vi "dfd_FXP Direct FIR with IS.vi"(6 "state in":i64[](array[numeric]), 7 "FXPOPs":T5[](array[typedef]) {"source" items=["Coef a/k"=0, "Coef b/v"=7, "Input"=1, "Output"=2, "Multiplicand"=3, "Product"=4, "Sum"=5, "Delay"=6, "Gain"=8]}, 8 "filtering statistics in":T4(array[cluster]) {"statistics information"."min value" format="%.2f"; "statistics information"."max value" format="%.2f"; "Quantizer Source" items=["Coefficients a/k"=0, "Coefficients b/v"=7, "Input"=1, "Output"=2, "Multiplicand"=3, "Product"=4, "Sum"=5, "Delay"=6]}, 10 "coef b":T7, 11 "X":T7) -> (0 "filtering statistics out":T4(array[cluster]) {"statistics information"."min value" format="%.2f"; "statistics information"."max value" format="%.2f"; "Quantizer Source" items=["Coefficients a/k"=0, "Coefficients b/v"=7, "Input"=1, "Output"=2, "Multiplicand"=3, "Product"=4, "Sum"=5, "Delay"=6]}, 3 "filtered X":T7, 4 "state out":i64[](array[numeric]))   [LabVIEW 2017, in "NI_DigFilter_FXP.lvlib"]
uses:
  <vilib>/addons/Digital Filter Design/NI_DigFilter_FXP.lvlib
  <vilib>/addons/Digital Filter Design/_Objects.llb/dfd_DFXP Data Type (vector).ctl
  <vilib>/addons/Digital Filter Design/_Objects.llb/dfd_DFXP Operation Parameter.ctl
  <vilib>/addons/Digital Filter Design/_Objects.llb/dfd_Internal Quantization Srcs.ctl
  <vilib>/addons/Digital Filter Design/_Objects.llb/DFD Quantization Sources.ctl
  <vilib>/addons/Digital Filter Design/_Objects.llb/DFD FXP Statistics Data.ctl
  <vilib>/addons/Digital Filter Design/_Objects.llb/dfd_DFXP Data Type (scaler).ctl
  <vilib>/addons/Digital Filter Design/NI_DigFilterLicensed.lvlib
panel:
  in  "DFXP Value":T1={"value"=0, "wl"=0, "iwl"=0, "Signed"=TRUE} {"value" format="%.0x"}
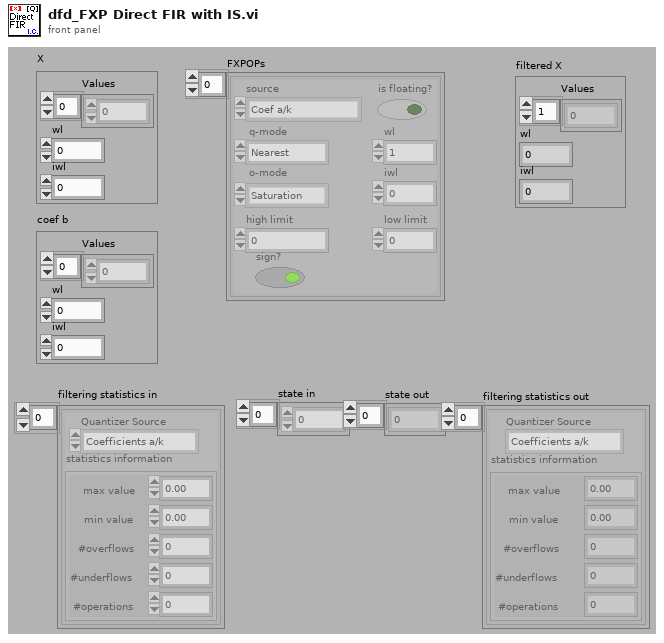
[diagram p1: front panel]
types:
  T1 = typedef "dfd_DFXP Data Type (scaler).ctl" = cluster{"value":i64, "wl":i16, "iwl":i16, "Signed":bool}
  T2 = typedef "NI_DigFilterLicensed.lvlib/DFD Quantization Sources.ctl" = u16
  T3 = typedef "NI_DigFilterLicensed.lvlib/DFD FXP Statistics Data.ctl" = cluster{"max value":ext, "min value":ext, "#overflows":i32, "#underflows":i32, "#operations":i32}
  T4 = cluster{"Quantizer Source":T2, "statistics information":T3}[]
  T5 = typedef "dfd_DFXP Operation Parameter.ctl" = cluster{"source":T6, "is floating?":bool, "o-mode":enum16{"Saturation", "Wrap"}, "q-mode":enum16{"Nearest", "Truncation"}, "wl":i16, "high limit":i64, "low limit":i64, "iwl":i16, "sign?":bool}
  T6 = typedef "NI_DigFilterLicensed.lvlib/dfd_Internal Quantization Srcs.ctl" = u16
  T7 = typedef "dfd_DFXP Data Type (vector).ctl" = cluster{"Values":i64[], "wl":i16, "iwl":i16}
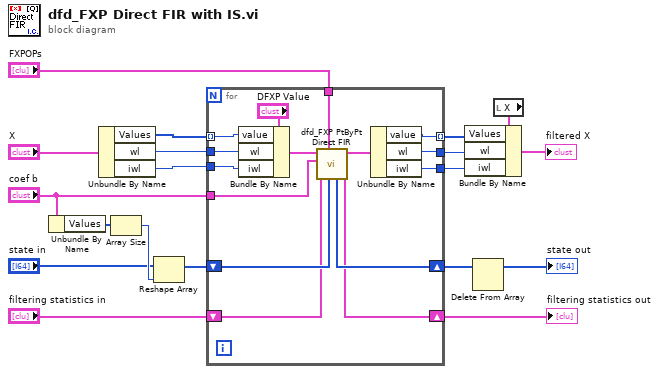
[diagram p0: block diagram]
diagram:
  n1 = Unbundle By Name("coef b") -> ("Values"=w13:i64[])
  n2 = Unbundle By Name("X") -> ("Values"=w8:i64[], "wl"=w7:i16, "iwl"=w6:i16)
  n3 = Array Size(array=w13) -> (size(s)=w15:i32)
  n4 = Reshape Array("state in", w15) -> (w19:i64[])
  n5 = for {
    tunnel: "coef b" -> [w34]
    shift-right: [w32] -> w18
    shift-left: w19 -> [w33]
    tunnel: [w22] -> w4 mode=indexing
    tunnel: "FXPOPs" -> [w30]
    shift-right: [w28] -> w16
    shift-left: "filtering statistics in" -> [w29]
    tunnel: w8 -> [w26] mode=indexing
    tunnel: w7 -> [w24]
    tunnel: w6 -> [w23]
    tunnel: [w21] -> w3
    tunnel: [w20] -> w2
    n6 = Bundle By Name(cluster="DFXP Value", "value"=w26, "wl"=w24, "iwl"=w23) -> (w25:T1)
    n7 = call <vilib>:"dfd_FXP PtByPt Direct FIR.vi"("state in"=w33, "FXPOPs"=w30, "filtering statistics in"=w29, "coef b"=w34, "x"=w25) -> ("filtering statistics out"=w28:T4, "filtered x"=w31:T1, "state out"=w32:i64[])  [unwired: 2 in, 2 out]
    n8 = Unbundle By Name(w31) -> ("value"=w22:i64, "wl"=w21:i16, "iwl"=w20:i16)
  }
  "filtering statistics out" <- w16
  n9 = Delete From Array(array=w18) -> (array with subset deleted=→"state out":i64[])  [unwired: 2 in, 1 out]
  n10 = local read "X"() -> (w5:T7)
  n11 = Bundle By Name(cluster=w5, "Values"=w4, "wl"=w3, "iwl"=w2) -> (→"filtered X":T7)
